vi "例程15-求稳定状态时的曲线.vi"() -> ()   [LabVIEW 2016]
panel:
  out "增长速度":dbl
  out "波形图":dbl[](graph)
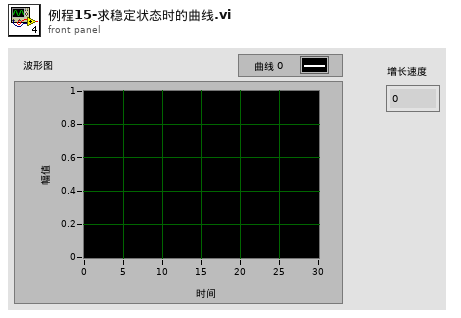
[diagram p1: front panel]
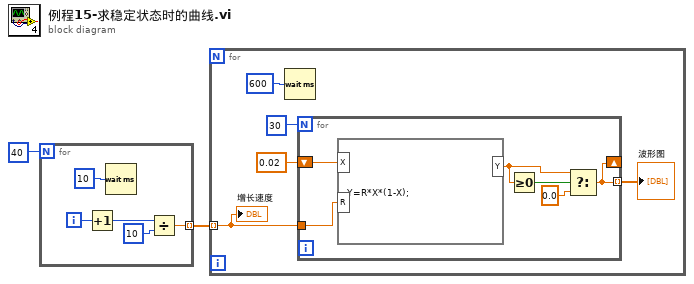
[diagram p0: block diagram]
diagram:
  n1 = for {
    N: 40 -> [_]
    tunnel: [w3] -> w1 mode=indexing
    i -> [w6]
    n2 = Increment(x=w6) -> (x+1=w5:i32)
    n3 = Wait (ms)(milliseconds to wait=u32 10 ("等待时间（毫秒）")) -> ()  [unwired: 1 out]
    n4 = Divide(x=w5, y=10) -> (x/y=w3:dbl)
  }
  n5 = for {
    tunnel: w1 -> [w8] mode=indexing
    n6 = Wait (ms)(milliseconds to wait=u32 600 ("等待时间（毫秒）")) -> ()  [unwired: 1 out]
    n7 = for {
      N: 30 -> [_]
      tunnel: [w14] -> w12 mode=indexing
      tunnel: w8 -> [w16]
      shift-right: [w14] -> _
      shift-left: 0.02 -> [w15]
      n8 = formula code="Y=R*X*(1-X);"("X"=w15, "R"=w16) -> ("Y"=w13:dbl)
      n9 = Greater Or Equal To 0?(x=w13) -> (x >= 0?=w18:bool)
      n10 = Select(t=w13, s=w18, f=0.0) -> (s? t:f=w14:dbl)
    }
    "波形图" <- w12
    "增长速度" <- w8
  }
